vi "Day 6.vi"() -> ()   [LabVIEW 2021]
panel:
  in  "Input File":enum32{"example input", "input"}(radio)
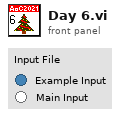
[diagram p1: front panel]
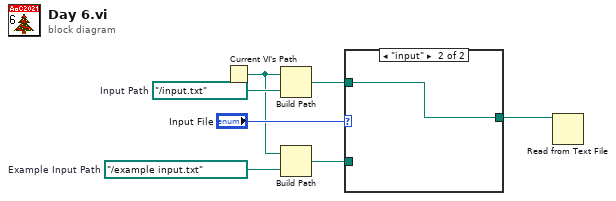
[diagram p0: block diagram]
diagram:
  w6 = path "../example input.txt"  # Example Input Path
  w7 = path "../input.txt"  # Input Path
  n1 = Current VI's Path() -> (path=w1:path)
  n2 = Build Path(base path=w1, name or relative path=w7) -> (appended path=w4:path)
  n3 = Build Path(base path=w1, name or relative path=w6) -> (appended path=w3:path)
  n4 = case shown="\"input\"" "Input File" {
    tunnel: w4 -> [_ w9]
    tunnel: w3 -> [w8 _]
    tunnel: [w8 w9] -> w2
    frame "example input" {
    }
    frame "input" {
    }
  }
  n5 = Read from Text File(file (use dialog)=w2) -> ()  [unwired: 3 in, 4 out]
